vi "new channel1553.vi"(6 "channel1553 configuration":T1={"channelBufferMaxSizeKB"=1024, "amplitudeAdjustEnable"=FALSE, "amplitudePercent"=50.0, "termination"=0, "modeCodes"=0, "broadcast"=FALSE} {"termination" items=["Off", "OnA", "OnB", "On"]; "modeCodes" items=["MC01", "MC1", "MC0", "None"]}, 7 "errorInjection configuration":T2 {"errorMessages" items=["Tagged", "Any"]; "state" items=["Off", "On", "Once", "External"]}, 8 "error in":errorcluster, 10 "hardwareChannel (-1)":i32=-1, 11 "name":string) -> (0 "error out":errorcluster, 3 "new channel1553":refnum<k24>)   [LabVIEW 2020, in "Ballard_1553_Hardware_ni.lvlib"]
uses:
  Ballard_1553_Hardware_ni.lvlib
  C:/Users/Administrator/Desktop/GIT/Ballard-MIL-STD-1553-Custom-Device/Source/System Explorer/SubVIs/Parse XML Ballard/1.2/BTIXML_SerDes.dll
  Ballard-MIL-STD-1553-Custom-Device/Source/System Explorer/SubVIs/Parse XML Ballard/1.2/BTIXML_SerDes.dll
  _typedefs/channel1553_errorInjection_type.ctl
  _typedefs/channel1553_type.ctl
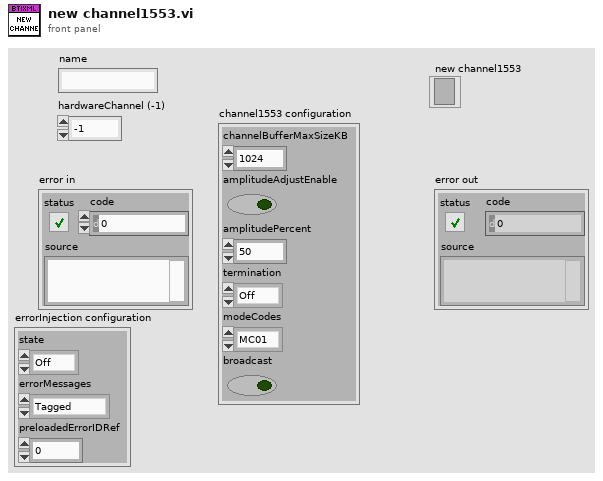
[diagram p1: front panel]
types:
  T1 = typedef "Ballard_1553_Hardware_ni.lvlib/channel1553_type.ctl" = cluster{"channelBufferMaxSizeKB":u32, "amplitudeAdjustEnable":bool, "amplitudePercent":dbl, "termination":i32, "modeCodes":i32, "broadcast":bool}
  T2 = typedef "Ballard_1553_Hardware_ni.lvlib/channel1553_errorInjection_type.ctl" = cluster{"state":i32, "errorMessages":i32, "preloadedErrorIDRef":i32}
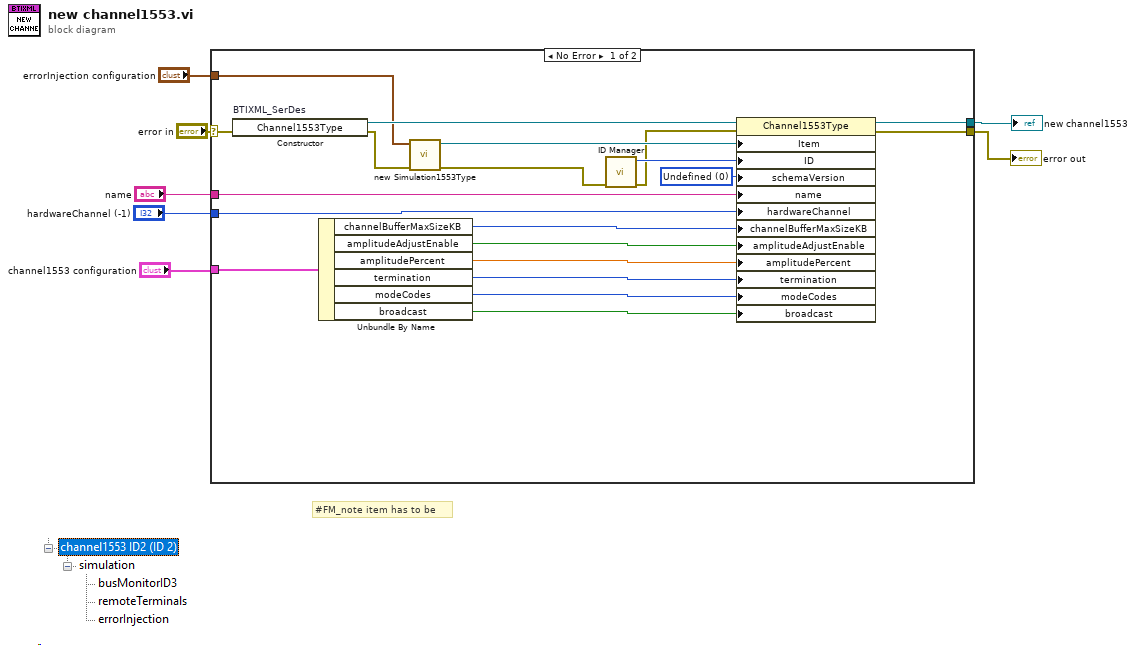
[diagram p0: block diagram]
diagram:
  # "#FM_note item has to be"
  n1 = case shown="No Error" "error in" {
    selector: "error in" -> [w27 w28]
    tunnel: [w25 w28] -> w6
    tunnel: [w24 _] -> w5
    tunnel: "name" -> [w23 _]
    tunnel: "hardwareChannel (-1)" -> [w22 _]
    tunnel: "channel1553 configuration" -> [w21 _]
    tunnel: "errorInjection configuration" -> [w11 _]
    frame No Error {
      w14 = 0 items=["Undefined", "Item10", "Item11", "Item12"] ("schemaVersion")
      n2 = constructor on="BTIXML_SerDes" class="Channel1553Type"(error in=w27) -> (reference out=w26:refnum<k24>, error out=w13:errorcluster)  [unwired: 2 in, 1 out]
      n3 = Unbundle By Name(w21) -> ("channelBufferMaxSizeKB"=w20:u32, "amplitudeAdjustEnable"=w19:bool, "amplitudePercent"=w18:dbl, "termination"=w17:i32, "modeCodes"=w16:i32, "broadcast"=w15:bool)
      n4 = call "new Simulation1553Type.vi"("error in"=w13, "errorInjection configuration"=w11) -> ("error out"=w10:errorcluster, "new Simulation1553Type"=w12:refnum<k24>)  [unwired: 8 in]
      n5 = call "ID Manager.vi"("error in"=w10) -> ("error out"=w8:errorcluster, "ID out"=w9:i32)  [unwired: 9 in]
      n6 = property class="Channel1553Type"(reference=w26, error in=w8, "Item"=w12, "ID"=w9, "schemaVersion"=w14, "name"=w23, "hardwareChannel"=w22, "channelBufferMaxSizeKB"=w20, "amplitudeAdjustEnable"=w19, "amplitudePercent"=w18, "termination"=w17, "modeCodes"=w16, "broadcast"=w15) -> (reference out=w24:refnum<k24>, error out=w25:errorcluster)
    }
    frame Error {
    }
  }
  "error out" <- w6
  "new channel1553" <- w5
